vi "c_Start Log.vi"() -> (1 "Case Label":T1)   [LabVIEW 2021, in "Maestro Data Logg.lvclass"]
uses:
  Maestro Data Logg.lvclass
  <vilib>/addons/_Workers/Library/Case Label.ctl
  <vilib>/addons/_Workers/Library/Workers.lvlib
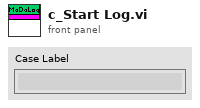
[diagram p1: front panel]
types:
  T1 = typedef "Workers.lvlib/Case Label.ctl" = string
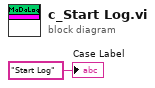
[diagram p0: block diagram]
diagram:
  "Case Label" <- T1 "Start Log" ("Case Label")
